vi "Unit Test.vi"() -> ()   [LabVIEW 2018]
uses:
  Thermocouple.lvclass
  Custom Controls/System Units.ctl
  Thermocouple.lvclass/Thermocouple.ctl
  Thermocouple.lvlib
panel:
  out "Temperature":dbl
  out "Thermocouple out":refnum<class "Thermocouple.lvclass">
  out "error out":errorcluster
  in  "SI":T1
  in  "error in (no error)":errorcluster
  in  "Resource":tag
  in  "Thermocouple in":refnum<class "Thermocouple.lvclass">
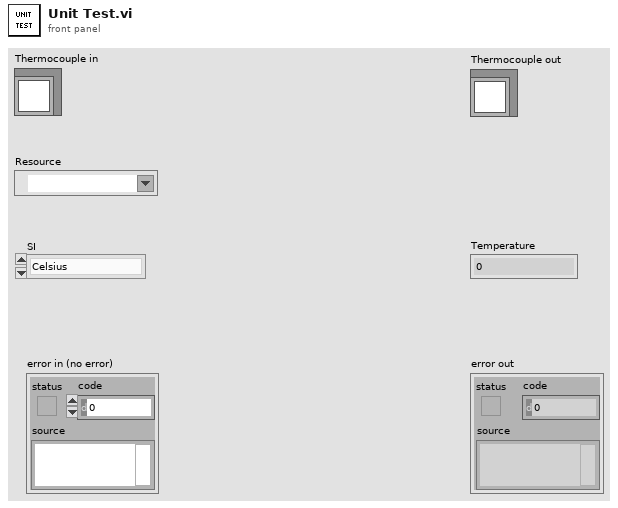
[diagram p1: front panel]
types:
  T1 = typedef "Thermocouple.lvlib/System Units.ctl" = enum16{"Celsius", "Fahrenheit"}
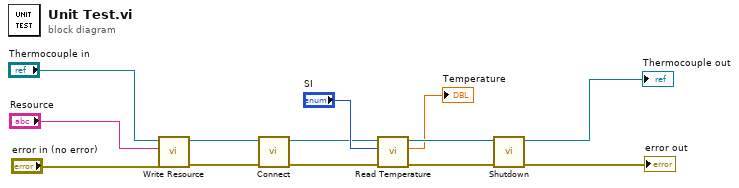
[diagram p0: block diagram]
diagram:
  n1 = call "Write Resource.vi"("error in (no error)"="error in (no error)", "Resource"="Resource", "Thermocouple in"="Thermocouple in") -> ("error out"=w4:errorcluster, "Thermocouple out"=w1:refnum<class "Thermocouple.lvclass">)  [unwired: 7 in]
  n2 = call-dynamic "Connect.vi"("error in (no error)"=w4, "Thermocouple in"=w1) -> ("error out"=w3:errorcluster, "Thermocouple out"=w2:refnum<class "Thermocouple.lvclass">)  [unwired: 8 in]
  n3 = call-dynamic "Read Temperature.vi"("error in (no error)"=w3, "SI"="SI", "Thermocouple in"=w2) -> ("error out"=w8:errorcluster, "Temperature"=→"Temperature":dbl, "Thermocouple out"=w9:refnum<class "Thermocouple.lvclass">)  [unwired: 6 in]
  n4 = call "Shutdown.vi"("error in (no error)"=w8, "Thermocouple in"=w9) -> ("error out"=→"error out":errorcluster, "Thermocouple out"=→"Thermocouple out":refnum<class "Thermocouple.lvclass">)  [unwired: 8 in]
